vi "citTemplate.sendAckNotifier.vi"(0 "notification data":string, 2 "notifierHandle in":T2, 11 "error in":errorcluster) -> ()   [LabVIEW 2016]
uses:
  citTemplate.notifierHandle.ctl
  citTemplate.notifierData.ctl
panel:
  in  "notifierData":T1
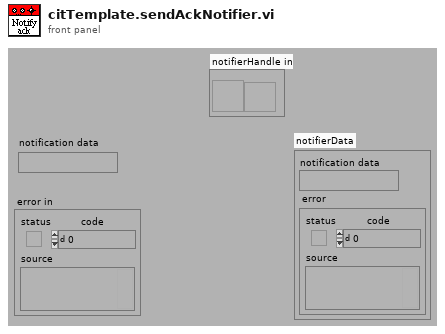
[diagram p1: front panel]
types:
  T1 = typedef "citTemplate.notifierData.ctl" = cluster{"notification data":string, "error":errorcluster}
  T2 = typedef "citTemplate.notifierHandle.ctl" = refnum<notifier>
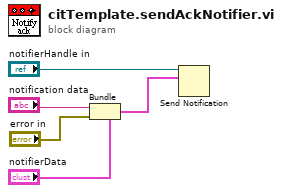
[diagram p0: block diagram]
diagram:
  n1 = Bundle(cluster="notifierData", "notification data"="notification data", "error"="error in") -> (w4:T1)
  n2 = Send Notification(notification=w4, notifier="notifierHandle in") -> ()  [unwired: 1 in, 2 out]
